vi "ReadFile.vi"   [LabVIEW 2021]
uses:
  Classes/ROFile/ROFile.lvclass
  Classes/RWFile/RWFile.lvclass
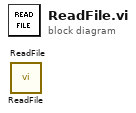
[diagram p0: block diagram]
diagram:
  n1 = call "ReadFile.vi"() -> ()  [unwired: 10 in, 2 out]
  n2 = call "ReadFile.vi"() -> ()  [unwired: 10 in, 2 out]
